vi "NI VeriStand - Unset Busy Cursor.vi"(8 "error in (no error)":errorcluster) -> (0 "error out":errorcluster)   [LabVIEW 2020, in "Custom Device API.lvlib"]
doc: "Releases the front panel cursor of the <B>System Explorer</B> window. Use this VI after a Page VI finishes initializing."
uses:
  <vilib>/NI VeriStand/Custom Device API/Custom Device API.lvlib
  fe84d860-e738-40fa-b85d-c9a3e67e9d6b.vi
  <vilib>/NI VeriStand/Custom Device API/Custom Device Offline Path.vi
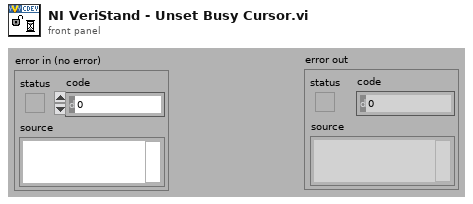
[diagram p1: front panel]
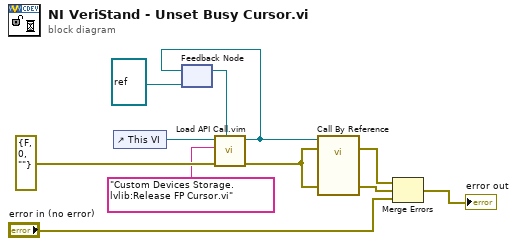
[diagram p0: block diagram]
diagram:
  n1 = control-ref of="This VI"() -> (w7:refnum<vi>)
  n2 = feedback #1(refnum<vi> refnum ("type specifier VI Refnum (for type only)")) -> (w8:refnum<vi>)
  n3 = call "Load API Call.vim"("VI reference in"=w8, "error in (no error)"=errorcluster {"status"=FALSE, "code"=0, "source"=""}, "VI qualified name"="Custom Devices Storage.lvlib:Release FP Cursor.vi", "Caller VI ref"=w7) -> ("error out"=w4:errorcluster, "VI reference"=w5:refnum<vi>)  [unwired: 6 in]
  n4 = feedback-in #1(w5) -> ()
  n5 = call-by-ref "?"(reference=w5, error in=w4, 8:"error in (no error)"=w4) -> (error out=w1:errorcluster, 0:"error out"=w11:errorcluster)  [unwired: 10 in, 1 out]
  n6 = Merge Errors(w1, w11, "error in (no error)") -> (→"error out":errorcluster)
